vi "Append Unicode Phrase.vi"(0 "PDF Report IN":refnum<class "PDF Report Class.lvclass">=refnum, 1 "Type (ASCII default)":enum16{"ASCII", "Unicode"}(ring), 2 "Phrase":string, 7 "Direction":enum16{"Default", "LTR", "No Bidi", "RTL"}(ring), 11 "error in (no error)":errorcluster, 12 "Font":T2={"Name"="", "Size"=-1.0, "Color"=0, "Style"={"Bold"=FALSE, "Italic"=FALSE, "Underline"=FALSE, "Strikeout"=FALSE}, "Type"={"Type&direction"=enum."Select", "Embedded"=FALSE, "Encoding"="CP1252"}}, 14 "Line spacing":T1) -> (4 "PDF Report OUT":refnum<class "PDF Report Class.lvclass">, 8 "x":u32, 15 "error out":errorcluster)   [LabVIEW 2019, in "Exaprom PDF.lvlib"]
doc: "Developed by Jean-Marc Simard\nCopyright © 2012, Exaprom Inc.\nAll rights reserved.\nLicense: BSD\n\nWith iTextSharp 4.1.6 (http://itextsharp.sourceforge.net)\nunder Mozilla Public License Version 1.1\n(http://www.mozilla.org/MPL/MPL-1.1.html)"
uses:
  Exaprom PDF.lvlib
  C:/work/niobrara_lv/labview pdf writer fixing/DLL/itextsharp.dll
  DLL/itextsharp.dll
  Controls/Text Controls/Texte alignement.ctl
  LV Class/Fonts Class/Font Class.lvclass
  LV Class/PDF Report Class/PDF Report Class.lvclass
  Controls/Font Controls/Font size.ctl
  Controls/Font Controls/Font color.ctl
  Controls/Text Controls/Line spacing.ctl
  Controls/Font Controls/Font complete cluster.ctl
  LV Class/Header and Footer Class/Header and Footer Class.lvclass
  Controls/Text Controls/Unicode/Type and run direction.ctl
  Controls/Font Controls/Type and encoding.ctl
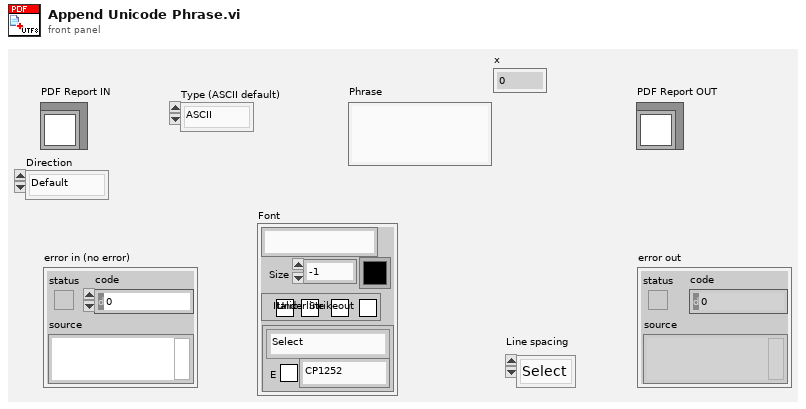
[diagram p1: front panel]
types:
  T1 = typedef "Exaprom PDF.lvlib/Line spacing.ctl" = enum16{"Select", "1.0", "1.5", "2.0"}
  T2 = typedef "Exaprom PDF.lvlib/Font complete cluster.ctl" = cluster{"Name":string, "Size":T3, "Color":T4, "Style":cluster{"Bold":bool, "Italic":bool, "Underline":bool, "Strikeout":bool}, "Type":T5}
  T3 = typedef "Exaprom PDF.lvlib/Font size.ctl" = sgl
  T4 = typedef "Exaprom PDF.lvlib/Font color.ctl" = u32
  T5 = typedef "Exaprom PDF.lvlib/Type and encoding.ctl" = cluster{"Type&direction":T6, "Embedded":bool, "Encoding":string}
  T6 = typedef "Exaprom PDF.lvlib/Type and run direction.ctl" = enum16{"Select", "ASCII", "UTF-16", "UTF-16 (default)", "UTF-16 (LTR)", "UTF-16 (RTL)"}
  T7 = typedef "Exaprom PDF.lvlib/Texte alignement.ctl" = enum16{"Select", "CENTER", "JUSTIFY", "LEFT", "RIGHT"}
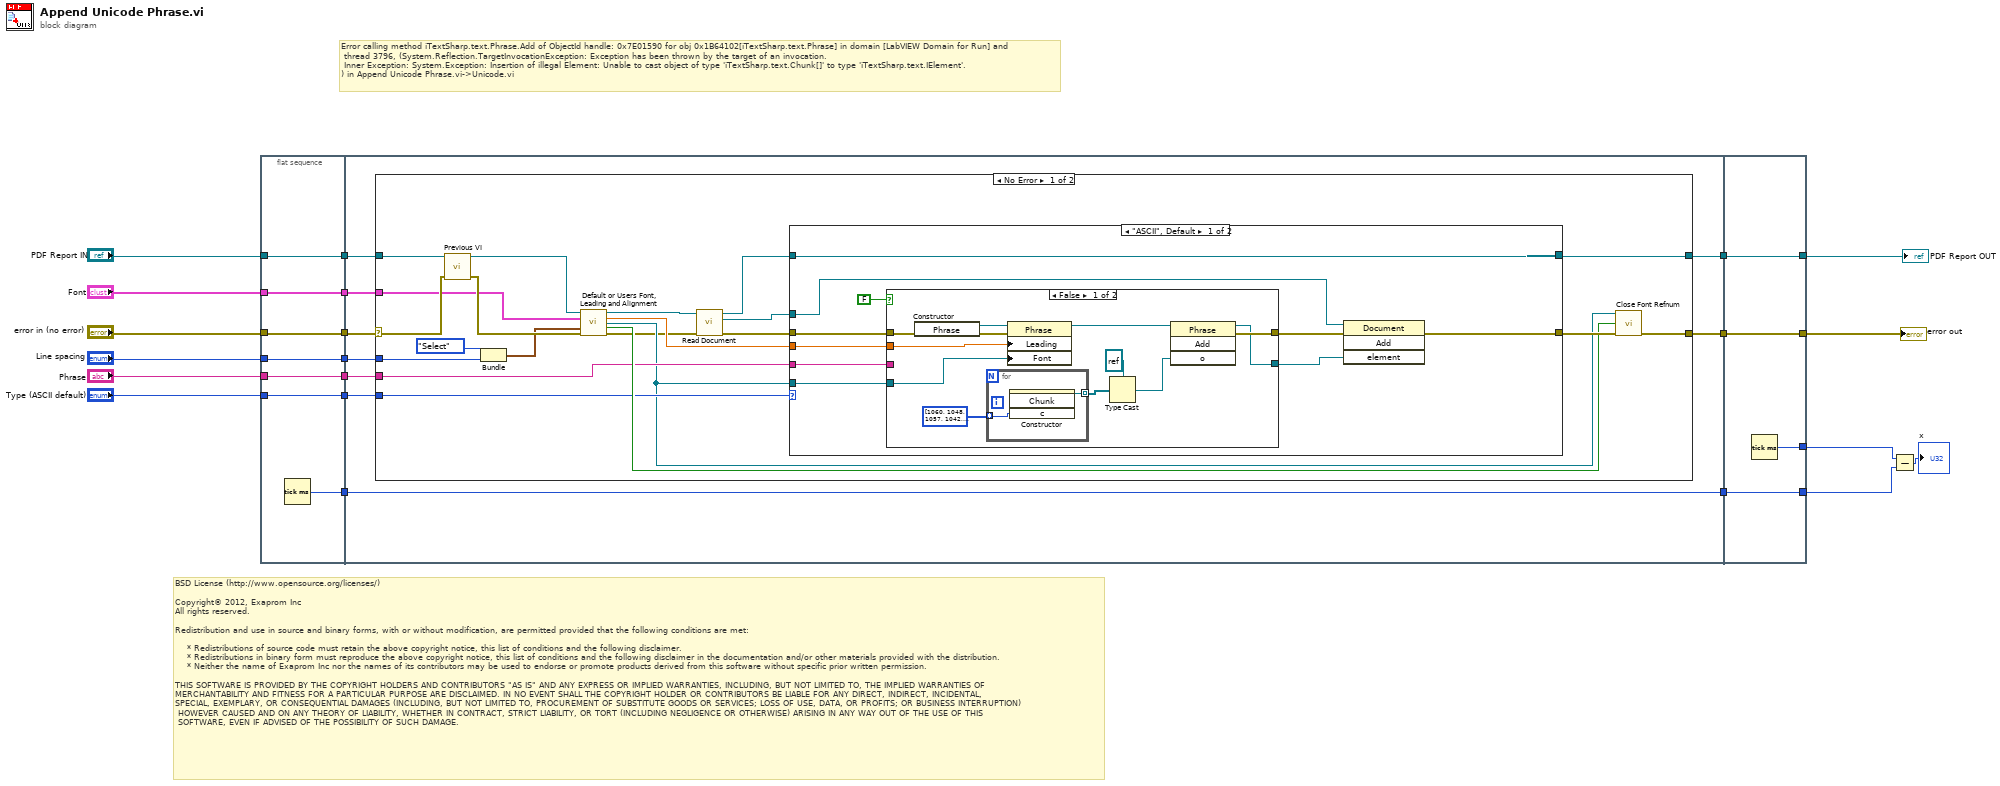
[diagram p0: block diagram]
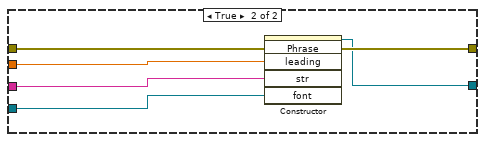
[diagram p2: hidden frame]
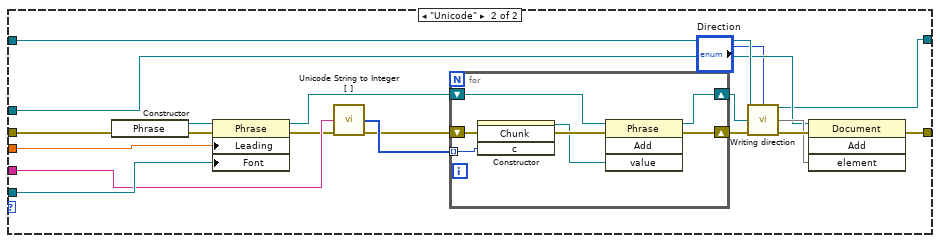
[diagram p3: hidden frame]
diagram:
  # "Error calling method iTextSharp.text.Phrase.Add of ObjectId handle: 0x7E01590 for obj 0x1B64102[iTextSharp.text.Phrase] in domain [LabVIEW Domain for Run] and\n thread 3796, (System.Reflection.TargetInvocationException: Exception has been thrown by the target of an invocation.\n\tInner Exception: System.Exception: Insertion of illegal Element: Unable to cast object of type 'iTextSharp.text.Chunk[]' to type 'iTextSharp.text.IElement'.\n) in Append Unicode Phrase.vi->Unicode.vi"
  # "BSD License (http://www.opensource.org/licenses/)\n\nCopyright© 2012, Exaprom Inc\nAll rights reserved.\n\nRedistribution and use in source and binary forms, with or without modification, are permitted provided that the following conditions are met:\n\n    * Redistributions of source code must retain the above copyright notice, this list of conditions and the following disclaimer.\n    * Redistributions in binary form must reproduce the above copyright notice, this list of conditions and the following disclaimer in the documentation and/or other materials provided with the distribution.\n    * Neither the name of Exaprom Inc nor the names of its contributors may be used to endorse or promote products derived from this software without specific prior written permission.\n\nTHIS SOFTWARE IS PROVIDED BY THE COPYRIGHT HOLDERS AND CONTRIBUTORS \"AS IS\" AND ANY EXPRESS OR IMPLIED WARRANTIES, INCLUDING, BUT NOT LIMITED TO, THE IMPLIED WARRANTIES OF \nMERCHANTABILITY AND FITNESS FOR A PARTICULAR PURPOSE ARE DISCLAIMED. IN NO EVENT SHALL THE COPYRIGHT HOLDER OR CONTRIBUTORS BE LIABLE FOR ANY DIRECT, INDIRECT, INCIDENTAL,\nSPECIAL, EXEMPLARY, OR CONSEQUENTIAL DAMAGES (INCLUDING, BUT NOT LIMITED TO, PROCUREMENT OF SUBSTITUTE GOODS OR SERVICES; LOSS OF USE, DATA, OR PROFITS; OR BUSINESS INTERRUPTION)\n HOWEVER CAUSED AND ON ANY THEORY OF LIABILITY, WHETHER IN CONTRACT, STRICT LIABILITY, OR TORT (INCLUDING NEGLIGENCE OR OTHERWISE) ARISING IN ANY WAY OUT OF THE USE OF THIS\n SOFTWARE, EVEN IF ADVISED OF THE POSSIBILITY OF SUCH DAMAGE."
  n1 = flat-sequence {
    tunnel: "Type (ASCII default)" -> [w23]
    tunnel: "Phrase" -> [w24]
    tunnel: "Line spacing" -> [w25]
    tunnel: "Font" -> [w26]
    tunnel: "error in (no error)" -> [w27]
    tunnel: "PDF Report IN" -> [w28]
    tunnel: [w28] -> w11
    tunnel: [w27] -> w10
    tunnel: [w26] -> w9
    tunnel: [w25] -> w8
    tunnel: [w24] -> w7
    tunnel: [w23] -> w6
    tunnel: [w22] -> w4
    tunnel: [w33] -> w13
    tunnel: [w32] -> w12
    tunnel: w11 -> [w37]
    tunnel: w10 -> [w36]
    tunnel: w9 -> [w35]
    tunnel: w8 -> [w34]
    tunnel: w7 -> [w31]
    tunnel: w6 -> [w30]
    tunnel: [w29] -> w5
    tunnel: w4 -> [w29]
    tunnel: [w118] -> w16
    tunnel: [w119] -> w17
    tunnel: w13 -> [w119]
    tunnel: w12 -> [w118]
    tunnel: [w117] -> w3
    tunnel: w5 -> [w117]
    tunnel: [w116] -> w2
    frame #0 {
      n2 = Tick Count (ms)() -> (millisecond timer value=w22:u32)
    }
    frame #1 {
      n3 = case shown="No Error" w36 {
        selector: w36 -> [w58 w115]
        tunnel: w35 -> [w45 _]
        tunnel: [w44 w114] -> w32
        tunnel: [w43 w115] -> w33
        tunnel: w37 -> [w56 w114]
        tunnel: w34 -> [w55 _]
        tunnel: w31 -> [w48 _]
        tunnel: w30 -> [w47 _]
        frame No Error {
          n4 = call "Previous VI.vi"("PDF Report IN"=w56, "error in (no error)"=w58) -> ("PDF Report OUT"=w52:refnum<class "PDF Report Class.lvclass">, "error out"=w57:errorcluster)  [unwired: 12 out]
          n5 = Bundle("Aligment"=Texte_alignement."Select", "Line spacing"=w55) -> (w54:cluster{"Aligment":T7, "Line spacing":T1})  [unwired: 1 out]
          n6 = call "Default or Users Font, Leading and Alignment.vi"("PDF Report"=w52, "Font"=w45, "Paragraphe cluster"=w54, "error in (no error)"=w57) -> ("PDF Report duplicate"=w40:refnum<class "PDF Report Class.lvclass">, "Leading"=w51:T3, "Font Ref"=w46:refnum<k24>, "Close Font Ref"=w49:bool, "error out"=w41:errorcluster)  [unwired: 1 in, 6 out]
          n7 = call-dynamic "Read Document.vi"("error in (no error)"=w41, "PDF Report Class in"=w40) -> ("error out"=w42:errorcluster, "Document"=w38:refnum<k24>, "PDF Report Class out"=w39:refnum<class "PDF Report Class.lvclass">)  [unwired: 7 in]
          n8 = case shown="\"ASCII\", Default" w47 {
            tunnel: w42 -> [w68 w103]
            tunnel: w51 -> [w67 w102]
            tunnel: [w62 w94] -> w50
            tunnel: w48 -> [w65 w100]
            tunnel: w46 -> [w66 w101]
            tunnel: [w61 w90] -> w44
            tunnel: w39 -> [w61 w92]
            tunnel: w38 -> [w60 w91]
            frame "ASCII", Default {
              n9 = case shown="False" FALSE {
                tunnel: w68 -> [w77 w88]
                tunnel: w67 -> [w74 w87]
                tunnel: w66 -> [w73 w86]
                tunnel: w65 -> [_ w85]
                tunnel: [w76 w84] -> w64
                tunnel: [w75 w83] -> w63
                frame False {
                  n10 = constructor class="Phrase"(error in=w77) -> (reference out=w78:refnum<k24>, error out=w79:errorcluster)  [unwired: 2 in, 1 out]
                  n11 = for {
                    tunnel: u16[] [1060, 1048, 1057, 1042, 1059, 1040, 1055, 1056, 1064, 1054, 1051, 1044, 1068, 1058, 1065, 1047, 1049, 1050, 1067, 1045, 1043, 1052, 1062, 1063, 1053, 1071] ("Integer [ ]") -> [w82] mode=indexing
                    tunnel: [w81] -> w72 mode=indexing
                    n12 = constructor class="Chunk"("c"=w82) -> (reference out=w81:refnum<k24>)  [unwired: 3 in, 3 out]
                  }
                  n13 = property class="Phrase"(reference=w78, error in=w79, "Leading"=w74, "Font"=w73) -> (reference out=w80:refnum<k24>)  [unwired: 1 out]
                  n14 = Type Cast(type=refnum<k24> refnum ("o"), x=w72) -> (*(type *) &x=w71:refnum<k24>)
                  n15 = invoke class="Phrase" method="Add"(reference=w80, "o"=w71) -> (reference out=w75:refnum<k24>, error out=w76:errorcluster)  [unwired: 2 in, 2 out]
                }
                frame True {
                  n16 = constructor class="Phrase"(error in=w88, "leading"=w87, "str"=w85, "font"=w86) -> (reference out=w83:refnum<k24>, error out=w84:errorcluster)  [unwired: 2 in, 4 out]
                }
              }
              n17 = invoke class="Document" method="Add"(reference=w60, error in=w64, "element"=w63) -> (error out=w62:errorcluster)  [unwired: 1 in, 3 out]
            }
            frame "Unicode" {
              n18 = constructor class="Phrase"(error in=w103) -> (reference out=w104:refnum<k24>, error out=w105:errorcluster)  [unwired: 2 in, 1 out]
              n19 = property class="Phrase"(reference=w104, error in=w105, "Leading"=w102, "Font"=w101) -> (reference out=w106:refnum<k24>, error out=w97:errorcluster)
              n20 = call "Unicode String to Integer [ ].vi"("Unicode String"=w100, "error in (no error)"=w97) -> ("Char U16 [ ]"=w99:u16[], "error duplicate"=w98:errorcluster)  [unwired: 11 in, 1 out]
              n21 = for {
                shift-right: [w112] -> w96
                shift-left: w106 -> [w113]
                shift-right: [w111] -> w107
                shift-left: w98 -> [w110]
                tunnel: w99 -> [w108] mode=indexing
                n22 = constructor class="Chunk"("c"=w108) -> (reference out=w109:refnum<k24>)  [unwired: 3 in, 3 out]
                n23 = invoke class="Phrase" method="Add"(reference=w113, error in=w110, "value"=w109) -> (reference out=w112:refnum<k24>, error out=w111:errorcluster)  [unwired: 1 in, 2 out]
              }
              n24 = call "Writing direction.vi"("PDF Report IN"=w92, "Text type"="Direction", "Paragraph refnum"=w96, "error in (no error)"=w107) -> ("PDF Report OUT"=w90:refnum<class "PDF Report Class.lvclass">, 8:w93, "error out"=w95:errorcluster)  [unwired: 9 in]
              n25 = invoke class="Document" method="Add"(reference=w91, error in=w95, "element"=w93) -> (error out=w94:errorcluster)  [unwired: 1 in, 3 out]
            }
          }
          n26 = call "Close Font Refnum.vi"("Font Refnum"=w46, "Close ?"=w49, "error in (no error)"=w50) -> ("error out"=w43:errorcluster)  [unwired: 12 in]
        }
        frame Error {
        }
      }
    }
    frame #2 {
      n27 = Tick Count (ms)() -> (millisecond timer value=w116:u32)
    }
  }
  n28 = Subtract(x=w2, y=w3) -> (x-y=→"x":u32)
  "PDF Report OUT" <- w16
  "error out" <- w17
